vi "DeleteCalibration.vi"(8 "error in (no error)":errorcluster, 10 "ID":string, 11 "ByteGSWebAPI-V0 in":refnum<class "ByteGSWebAPI-V0.lvclass">) -> (0 "error out":errorcluster, 3 "ByteGSWebAPI-V0 out":refnum<class "ByteGSWebAPI-V0.lvclass">, 4 "body":string, 6 "headers":string)   [LabVIEW 2019, in "ByteGSWebAPI-V0.lvclass"]
uses:
  ByteGSWebAPI-V0.lvclass
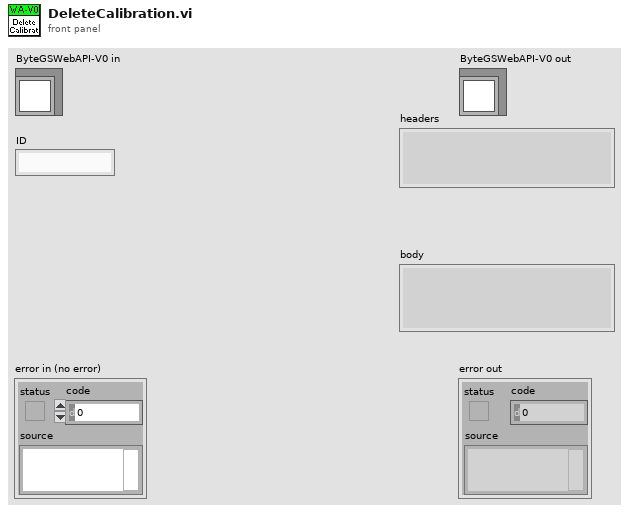
[diagram p1: front panel]
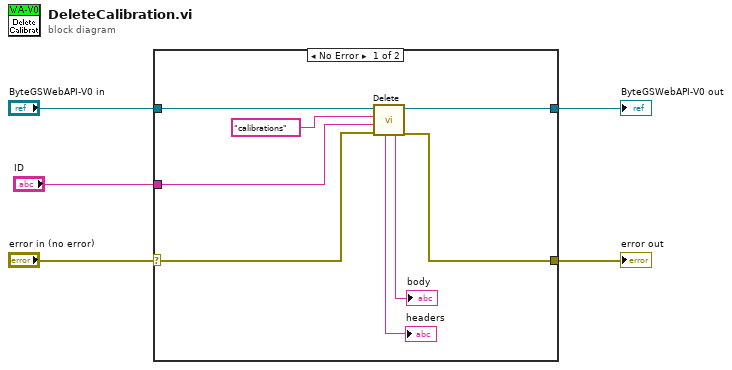
[diagram p0: block diagram]
diagram:
  n1 = case shown="No Error" "error in (no error)" {
    selector: "error in (no error)" -> [w9 w15]
    tunnel: [w6 w15] -> w4
    tunnel: [w13 w14] -> w2
    tunnel: "ByteGSWebAPI-V0 in" -> [w12 w14]
    tunnel: "ID" -> [w10 _]
    frame No Error {
      n2 = call-dynamic "Delete.vi"("error in (no error)"=w9, "Parameter"=w10, "Request"="calibrations", "ByteGSWebAPI-V0 in"=w12) -> ("error out"=w6:errorcluster, "ByteGSWebAPI-V0 out"=w13:refnum<class "ByteGSWebAPI-V0.lvclass">, "body"=→"body":string, "headers"=→"headers":string)  [unwired: 4 in]
    }
    frame Error {
    }
  }
  "error out" <- w4
  "ByteGSWebAPI-V0 out" <- w2
